vi "Host-Convert-U64-Complex.vi"(11 "Array in":u64[](array[numeric])) -> (3 "Array out":csg[](array[numeric]))   [LabVIEW 2015]
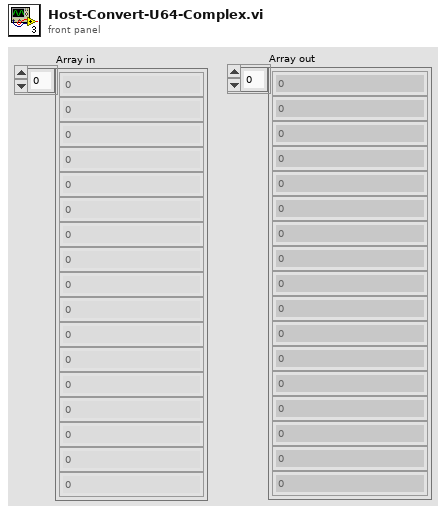
[diagram p1: front panel]
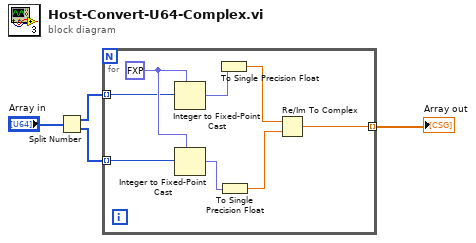
[diagram p0: block diagram]
diagram:
  n1 = Split Number(x="Array in") -> (hi(x)=w1:u32[], lo(x)=w2:u32[])
  n2 = for {
    tunnel: w1 -> [w10] mode=indexing
    tunnel: w2 -> [w11] mode=indexing
    tunnel: [w5] -> w3 mode=indexing
    w12 = fxp<+/-,32,12> 0.0 ("real data in")
    n3 = Integer to Fixed-Point Cast(fixed-point type=w12, integer=w10) -> (fixed-point=w8:fxp<+/-,32,12>)
    n4 = Integer to Fixed-Point Cast(fixed-point type=w12, integer=w11) -> (fixed-point=w9:fxp<+/-,32,12>)
    n5 = To Single Precision Float(number=w8) -> (single precision float=w7:sgl)
    n6 = To Single Precision Float(number=w9) -> (single precision float=w6:sgl)
    n7 = Re/Im To Complex(1:w6, 2:w7) -> (0:w5:csg)
  }
  "Array out" <- w3
